vi "Enable Timer.vi"(8 "error in (no error)":errorcluster, 9 "Enable Timer (T: Enable)":bool=TRUE, 10 "Channel (0: 30V Channel)":T1 caption="Channel (0: +6V)" items=["30V/3A Channel", "30V/3A Channel", "5V/3A Channel"], 11 "VISA resource name":refnum<visa-resource-name>) -> (0 "error out":errorcluster, 3 "VISA resource name out":refnum<visa-resource-name>)   [LabVIEW 2020, in "RIGOL DP800 Series.lvlib"]
doc: "Enables or disables the output timer."
uses:
  <instrlib>/RIGOL DP800 Series/RIGOL DP800 Series.lvlib
  <instrlib>/RIGOL DP800 Series/Public/Channels.ctl
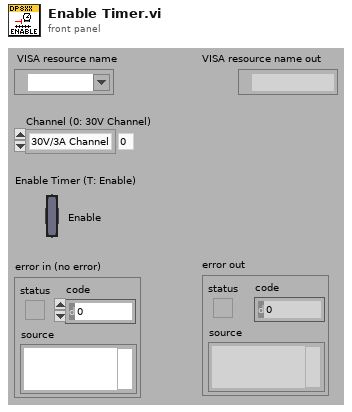
[diagram p1: front panel]
types:
  T1 = typedef "RIGOL DP800 Series.lvlib/Channels.ctl" = i32
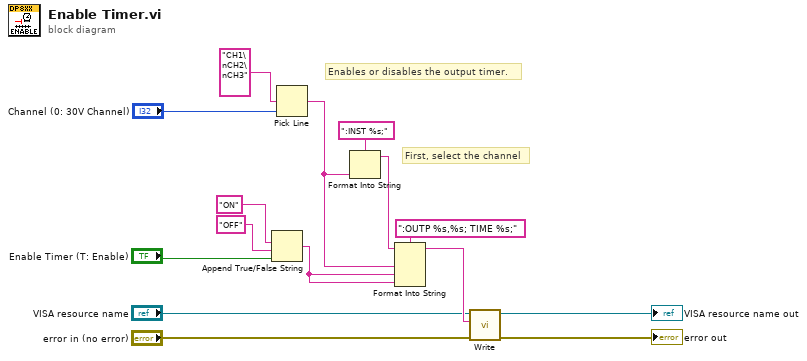
[diagram p0: block diagram]
diagram:
  # "First, select the channel"
  # "Enables or disables the output timer."
  n1 = Append True/False String(1:"Enable Timer (T: Enable)", 2:"OFF", 3:"ON") -> (0:w3:string)  [unwired: 1 out]
  n2 = Pick Line(multi-line string="CH1\nCH2\nCH3", line index="Channel (0: 30V Channel)") -> (output string=w1:string)  [unwired: 1 out]
  n3 = Format Into String(format string=":INST %s;", w1) -> (resulting string=w2:string)  [unwired: 2 in, 1 out]
  n4 = Format Into String(format string=":OUTP %s,%s; TIME %s;", initial string=w2, w1, w3, w3) -> (resulting string=w7:string)  [unwired: 1 in, 1 out]
  n5 = call <instrlib>:"Write.vi"("error in (no error)"="error in (no error)", "Write Buffer (\"\")"=w7, "VISA resource name"="VISA resource name") -> ("error out"=→"error out":errorcluster, "VISA resource name out"=→"VISA resource name out":refnum<visa-resource-name>)  [unwired: 7 in]
